vi "Lab2 - MatLab - Ines.vi"() -> ()   [LabVIEW 2025]
panel:
  out "Y vs. X":cluster{"Y":dbl[], "Y":dbl[]}[](graph)
  out "T vs. Y Position":cluster{"Y":dbl[], "Y":dbl[]}[](graph)
  out "T vs. X position":cluster{"Y":dbl[], "Y":dbl[]}[](graph)
  in  "Add Run":bool
  in  "Initial height (m)":dbl min=0.0
  in  "Initial speed (m/s":dbl=1.0 min=1.0
  in  "Angle (degrees)":dbl=1.0 min=1.0 max=89.0
  # "Ines Front Pannel"
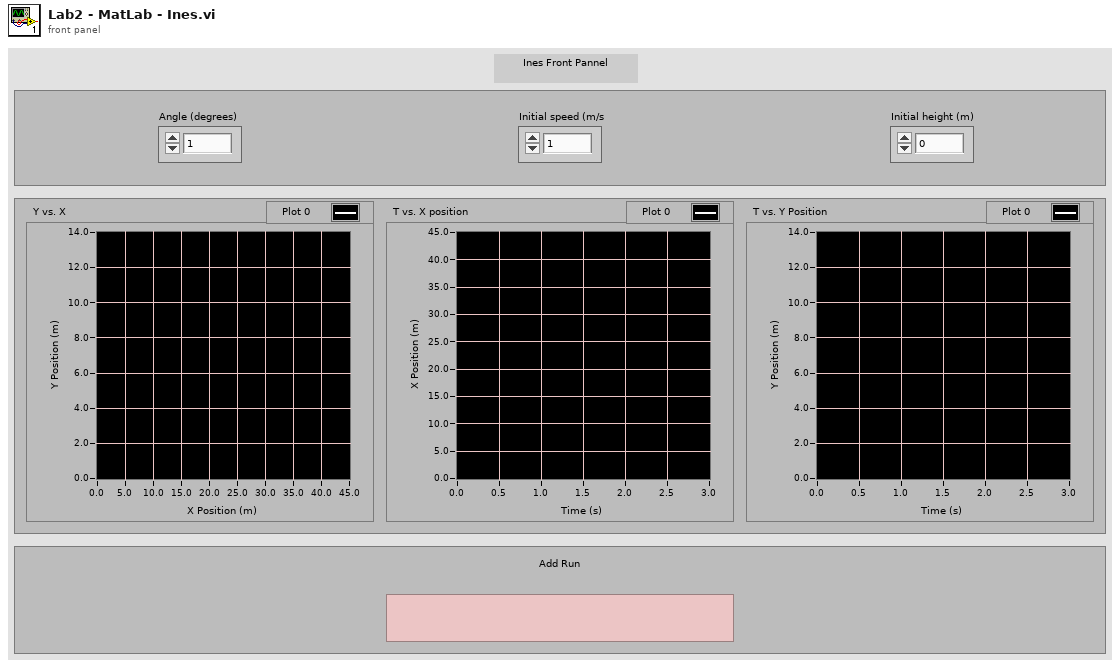
[diagram p1: front panel]
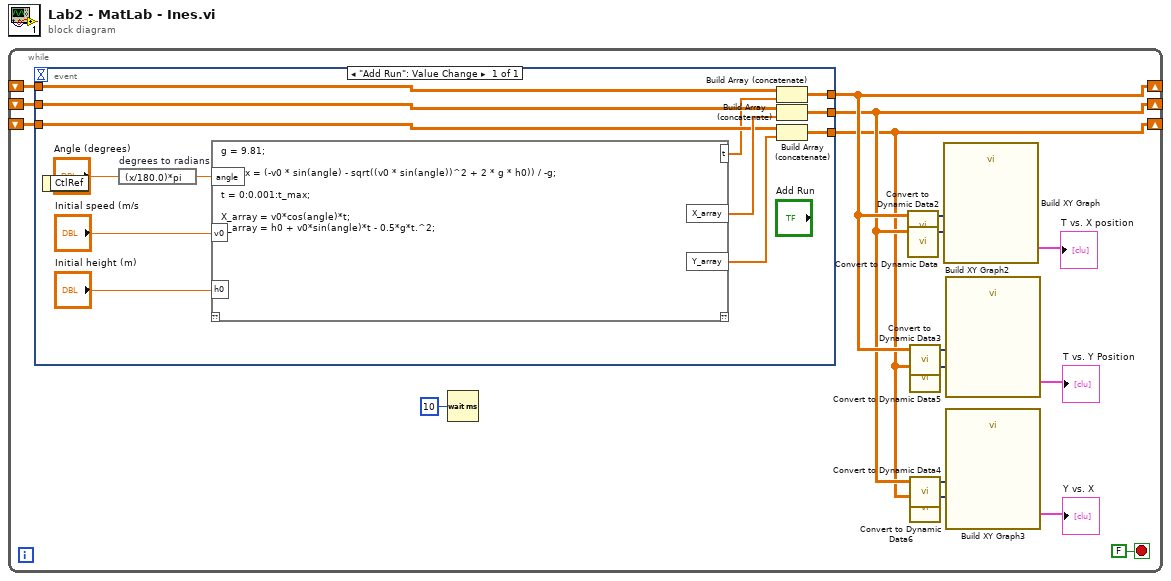
[diagram p0: block diagram]
diagram:
  n1 = while {
    shift-right: [w5] -> _
    shift-left: _ -> [w15]
    shift-right: [w2] -> _
    shift-left: _ -> [w14]
    shift-right: [w7] -> _
    shift-left: _ -> [w13]
    stop <- FALSE stop-if-true
    n2 = event shown="[0] \"Add Run\": Value Change" {
      selector: _ -> [_]
      dyn-events: _ -> [_]
      timeout: _ -> [_]
      tunnel: [w26] -> w5
      tunnel: w15 -> [w25]
      tunnel: [w23] -> w2
      tunnel: w14 -> [w22]
      tunnel: [w20] -> w7
      tunnel: w13 -> [w19]
      event "Add Run": Value Change {
        n3 = event-data() -> ()  [unwired: 1 in, 1 out]
        n4 = expression code="(x/180.0)*pi" "degrees to radians"("Angle (degrees)") -> (w30:dbl)
        n5 = script code="g = 9.81;\n\nt_max = (-v0 * sin(angle) - sqrt((v0 * sin(angle))^2 + 2 * g * h0)) / -g;\n\nt = 0:0.001:t_max;\n\nX_array = v0*cos(angle)*t;\nY_array = h0 + v0*sin(angle)*t - 0.5*g*t.^2;"("angle"=w30, "v0"="Initial speed (m/s", "h0"="Initial height (m)") -> ("X_array"=w27:dbl[], "Y_array"=w24:dbl[], "t"=w21:dbl[])  [unwired: 1 in, 1 out]
        n6 = Build Array (concatenate)(w19, w21) -> (w20:dbl[][])
        n7 = Build Array (concatenate)(w25, w27) -> (w26:dbl[][])
        n8 = Build Array (concatenate)(w22, w24) -> (w23:dbl[][])
      }
    }
    n9 = Wait (ms)(milliseconds to wait=u32 10) -> ()  [unwired: 1 out]
    n10 = call "Convert to Dynamic Data2"("2D Array"=w7) -> ("Dynamic Data Type"=w10:dynamicdata)  [unwired: 3 in]
    n11 = call "Convert to Dynamic Data"("2D Array"=w5) -> ("Dynamic Data Type"=w11:dynamicdata)  [unwired: 3 in]
    n12 = call "Convert to Dynamic Data3"("2D Array"=w7) -> ("Dynamic Data Type"=w6:dynamicdata)  [unwired: 3 in]
    n13 = call "Convert to Dynamic Data5"("2D Array"=w2) -> ("Dynamic Data Type"=w3:dynamicdata)  [unwired: 3 in]
    n14 = call "Convert to Dynamic Data4"("2D Array"=w5) -> ("Dynamic Data Type"=w4:dynamicdata)  [unwired: 3 in]
    n15 = call "Convert to Dynamic Data6"("2D Array"=w2) -> ("Dynamic Data Type"=w1:dynamicdata)  [unwired: 3 in]
    n16 = call "Build XY Graph"("Y Input"=w11, "X Input"=w10) -> ("XY Graph"=→"T vs. X position":cluster{"X":dbl[], "Y":dbl[]}[])  [unwired: 8 in, 1 out]
    n17 = call "Build XY Graph2"("Y Input"=w3, "X Input"=w6) -> ("XY Graph"=→"T vs. Y Position":cluster{"X":dbl[], "Y":dbl[]}[])  [unwired: 8 in, 1 out]
    n18 = call "Build XY Graph3"("Y Input"=w1, "X Input"=w4) -> ("XY Graph"=→"Y vs. X":cluster{"X":dbl[], "Y":dbl[]}[])  [unwired: 8 in, 1 out]
  }
